vi "DOE Dryer EF Data.vi"(8 "Error In":errorcluster, 11 "Dryer Initial IMC Data In":T1 {"Maximum Weight (lbf)" format="%03_6g"; "Average Weight (lbf)" format="%03_6g"; "Minimum Weight (lbf)" format="%03_6g"; "CEF (lbf/kWh)" format="%03_6g"; "Actual Final RMC (%)" format="%03_6g"; "Tolerance(%)" format="%0#_6g"; "Bone Dry Wt(lbs)" format="%03_6g"; "RMC (Desired %)" format="%0#_6g"; "Actual Initial RMC (%)" format="%03_6g"; "Measured IMC (lbs)" format="%0#_6g"}) -> (0 "Error Out":errorcluster, 2 "RMC Data":string[][](array[string]), 3 "Dryer Initial IMC Data out":T1 {"Maximum Weight (lbf)" format="%03_6g"; "Average Weight (lbf)" format="%03_6g"; "Minimum Weight (lbf)" format="%03_6g"; "CEF (lbf/kWh)" format="%03_6g"; "Actual Final RMC (%)" format="%03_6g"; "Tolerance(%)" format="%0#_6g"; "Bone Dry Wt(lbs)" format="%03_6g"; "RMC (Desired %)" format="%0#_6g"; "Actual Initial RMC (%)" format="%03_6g"; "Measured IMC (lbs)" format="%0#_6g"})   [LabVIEW 2019]
uses:
  Utility/Save File/File Setup (Public)/Type Definition/DPT IMC Data.ctl
  Type Definitions/DOE Dryer Standard.ctl
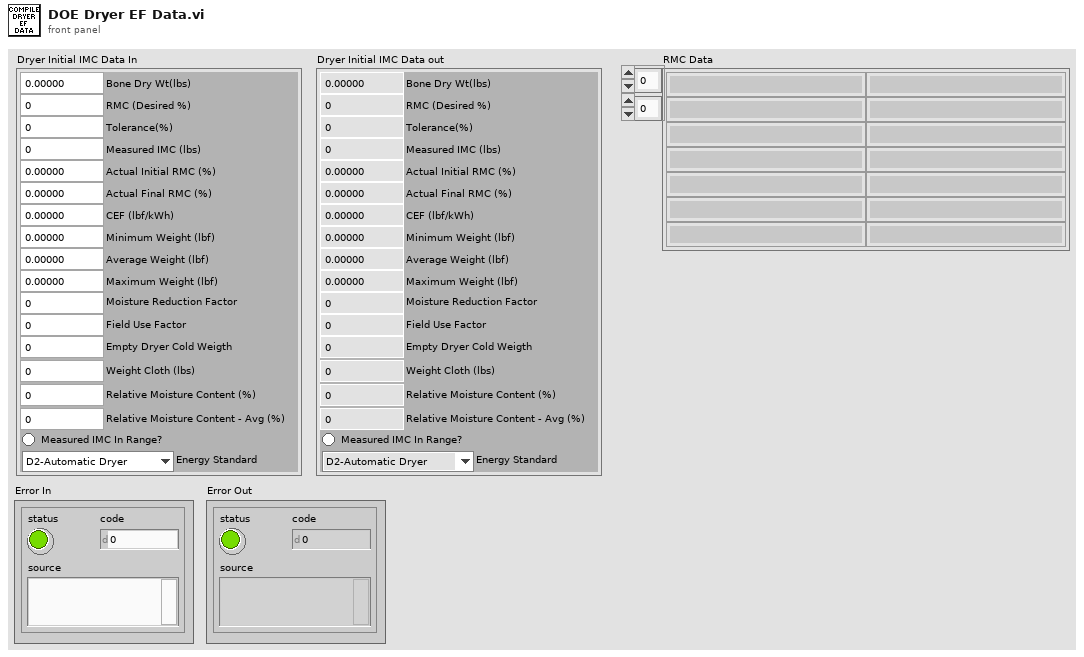
[diagram p1: front panel]
types:
  T1 = typedef "DPT IMC Data.ctl" = cluster{"Measured IMC (lbs)":dbl, "Actual Initial RMC (%)":dbl, "RMC (Desired %)":dbl, "Bone Dry Wt(lbs)":dbl, "Tolerance(%)":dbl, "Actual Final RMC (%)":dbl, "CEF (lbf/kWh)":dbl, "Minimum Weight (lbf)":dbl, "Average Weight (lbf)":dbl, "Maximum Weight (lbf)":dbl, "Measured IMC In Range?":bool, "Moisture Reduction Factor":dbl, "Field Use Factor":dbl, "Empty Dryer Cold Weigth":dbl, "Energy Standard":T2, "Weight Cloth (lbs)":dbl, "Relative Moisture Content (%)":dbl, "Relative Moisture Content - Avg (%)":dbl}
  T2 = typedef "DOE Dryer Standard.ctl" = enum16{"D2-Automatic Dryer", "D2-Timer Dryer", "D1-Automatic Dryer", "D1-Timer Dryer", "Other"}
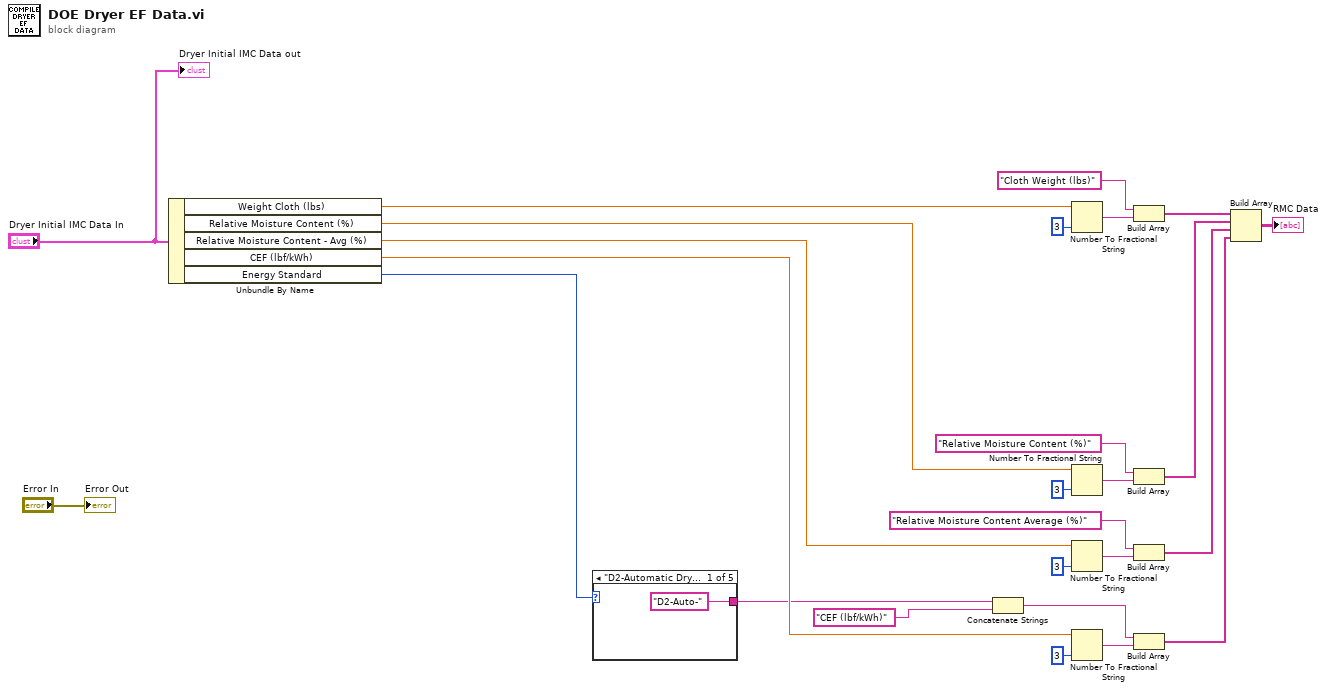
[diagram p0: block diagram]
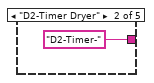
[diagram p2: hidden frame]
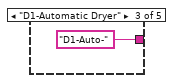
[diagram p3: hidden frame]
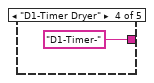
[diagram p4: hidden frame]
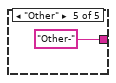
[diagram p5: hidden frame]
diagram:
  n1 = Unbundle By Name("Dryer Initial IMC Data In") -> ("Weight Cloth (lbs)"=w10:dbl, "Relative Moisture Content (%)"=w9:dbl, "Relative Moisture Content - Avg (%)"=w8:dbl, "CEF (lbf/kWh)"=w7:dbl, "Energy Standard"=w4:T2)
  n2 = case shown="\"D2-Automatic Dryer\", Default" w4 {
    tunnel: ["D2-Auto-" "D2-Timer-" "D1-Auto-" "D1-Timer-" "Other-"] -> w3
    frame "D2-Automatic Dryer", Default {
    }
    frame "D2-Timer Dryer" {
    }
    frame "D1-Automatic Dryer" {
    }
    frame "D1-Timer Dryer" {
    }
    frame "Other" {
    }
  }
  n3 = Concatenate Strings(w3, "CEF (lbf/kWh)") -> (w1:string)
  n4 = Number To Fractional String(number=w10, precision (6)=i16 3) -> (F-format string=w16:string)  [unwired: 2 in]
  n5 = Number To Fractional String(number=w9, precision (6)=i16 3) -> (F-format string=w12:string)  [unwired: 2 in]
  n6 = Number To Fractional String(number=w8, precision (6)=i16 3) -> (F-format string=w20:string)  [unwired: 2 in]
  n7 = Number To Fractional String(number=w7, precision (6)=i16 3) -> (F-format string=w24:string)  [unwired: 2 in]
  n8 = Build Array("Cloth Weight (lbs)", w16) -> (w18:string[])
  n9 = Build Array("Relative Moisture Content (%)", w12) -> (w17:string[])
  n10 = Build Array("Relative Moisture Content Average (%)", w20) -> (w22:string[])
  n11 = Build Array(w1, w24) -> (w25:string[])
  n12 = Build Array(w18, w17, w22, w25) -> (→"RMC Data":string[][])
  "Error Out" <- "Error In"
  "Dryer Initial IMC Data out" <- "Dryer Initial IMC Data In"
